vi "Is Alert Trigger.vi"(8 "times":dbl=5.0, 9 "standard deviation":dbl, 10 "mean":dbl, 11 "value":dbl) -> (3 "is alert?":bool)   [LabVIEW 2012]
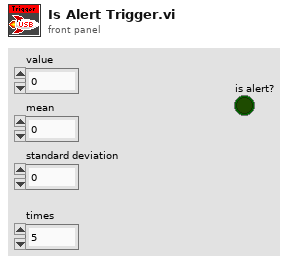
[diagram p1: front panel]
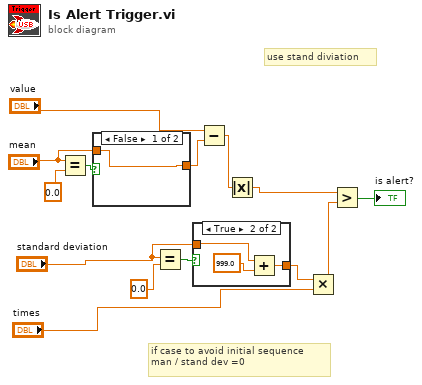
[diagram p0: block diagram]
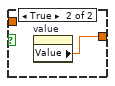
[diagram p2: hidden frame]
diagram:
  # "if case to avoid initial sequence \nman / stand dev =0"
  # "use stand diviation"
  n1 = Equal?(x="mean", y=0.0) -> (x = y?=w4:bool)
  n2 = case shown="False" w4 {
    tunnel: [w15 w16] -> w3
    tunnel: "mean" -> [w15 _]
    frame False {
    }
    frame True {
      n3 = property on="value" class="DigNum (strict)"() -> ("Value"=w16:dbl)  [unwired: 2 in, 2 out]
    }
  }
  n4 = Equal?(x="standard deviation", y=0.0) -> (x = y?=w13:bool)
  n5 = case shown="True" w13 {
    tunnel: "standard deviation" -> [w17 w19]
    tunnel: [w17 w18] -> w12
    frame False {
    }
    frame True {
      n6 = Add(x=w19, y=999.0) -> (x+y=w18:dbl)
    }
  }
  n7 = Subtract(x="value", y=w3) -> (x-y=w11:dbl)
  n8 = Absolute Value(x=w11) -> (abs(x)=w10:dbl)
  n9 = Multiply(x=w12, y="times") -> (x*y=w9:dbl)
  n10 = Greater?(x=w10, y=w9) -> (0:→"is alert?":bool)
